vi "ExtPRFCount.vi"(0 "Therapy Delay (ms)":dbl=1.0 min=2.5e-08 format="%.3f", 1 "Start Counter?":bool=TRUE, 9 "Divide prf by":i32=2, 11 "pulse width (s or cycles)":dbl=0.0001 min=2.5e-08 format="%.2e") -> (6 "Therapy Delay (ms) out":dbl format="%.2f", 15 "Divide prf out":i32=1)   [LabVIEW 2022 SP3]
uses:
  Motion Controllers/-MotionRoutines/MotionGlobals.vi
  <vilib>/DAQmx/create/channels.llb/DAQmx Create Channel (CO-Pulse Generation-Ticks).vi
  <vilib>/DAQmx/configure/timing.llb/DAQmx Timing (Implicit).vi
  Pulsers/PulserGlobals.vi
panel:
  out "pulse width (s or cycles) out":dbl format="%.2e"
  # "Indicates if counter 0 is is giving a 1-1 output pulse\n for each motor inpute or if it is generating a continous prf."
  # "Determines whether counter 1 is used to fire \ntherapy at some divided multiple of counter 0."
  # "Divide by two will stop unexpectadly because of the circuitry. Therefore can divide by\n1, then the next option is three"
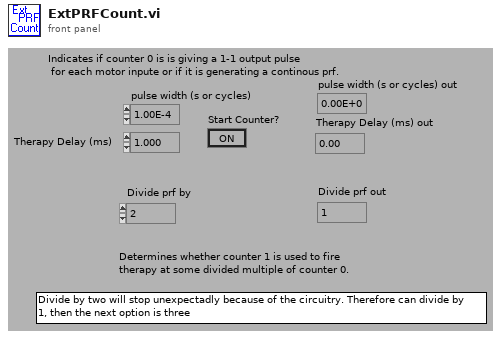
[diagram p1: front panel]
types:
  T1 = cluster{"Therapy frequency (MHz)":dbl, "Therapy amplitude (mV)":dbl, "time therapy on (s)":dbl, "Therapy Delay (ms) ":dbl, "Time (s)":dbl}
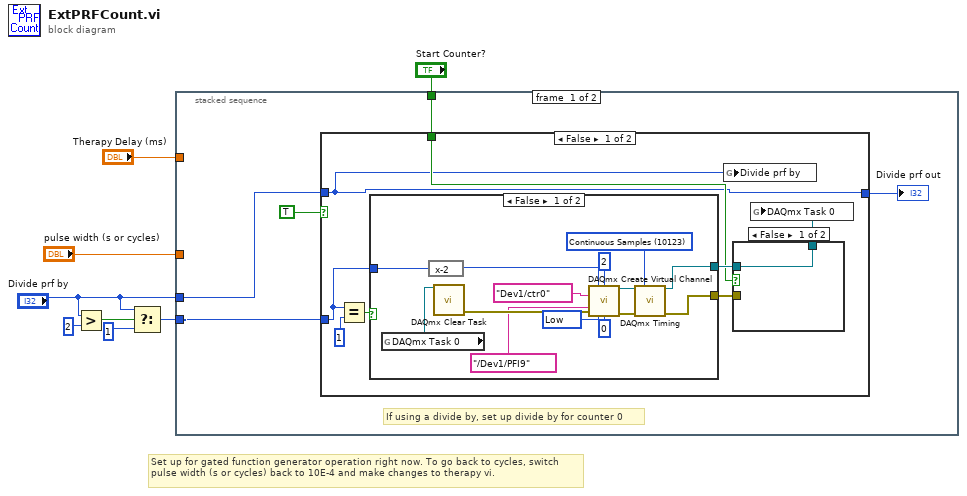
[diagram p0: block diagram]
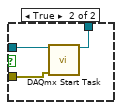
[diagram p2: hidden frame]
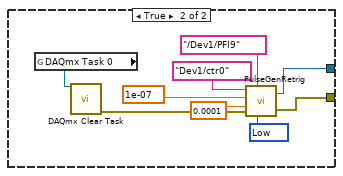
[diagram p3: hidden frame]
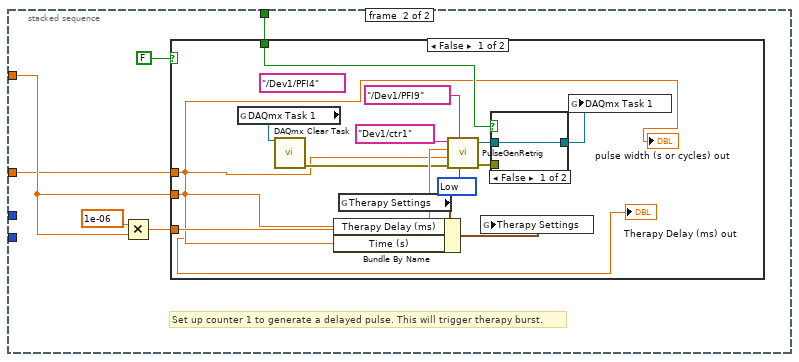
[diagram p5: hidden frame]
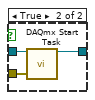
[diagram p6: hidden frame]
diagram:
  # "Set up for gated function generator operation right now. To go back to cycles, switch pulse width (s or cycles) back to 10E-4 and make changes to therapy vi."
  n1 = Greater?(x="Divide prf by", y=2) -> (0:w5:bool)
  n2 = Select(t="Divide prf by", s=w5, f=1) -> (s? t:f=w4:i32)
  n3 = stacked-sequence {
    tunnel: "Therapy Delay (ms)" -> [_ w54]
    tunnel: w4 -> [w12 _]
    tunnel: "Divide prf by" -> [w11 _]
    tunnel: "pulse width (s or cycles)" -> [_ w52]
    tunnel: "Start Counter?" -> [w9 w51]
    frame #0 {
      # "If using a divide by, set up divide by for counter 0"
      n4 = case shown="False" TRUE {
        tunnel: [w14 w49] -> w13
        tunnel: w11 -> [w14 _]
        tunnel: w12 -> [w19 w49]
        tunnel: w9 -> [w15 _]
        frame False {
          n5 = Equal?(x=w19, y=1) -> (x = y?=w20:bool)
          n6 = case shown="False" w20 {
            tunnel: w19 -> [w27 _]
            tunnel: [w39 w48] -> w18
            tunnel: [w38 w47] -> w17
            frame False {
              w29 = 10123 items=["Finite Samples"=10178, "Continuous Samples"=10123, "Hardware Timed Single Point"=12522] ("sample mode")
              w32 = 10214 items=["High"=10192, "Low"=10214] ("idle state")
              n7 = global read "MotionGlobals.vi" "DAQmx Task 0"() -> (w36:refnum<k21>)
              n8 = expression code="x-2"(w27) -> (w26:i32)
              n9 = call <vilib>:"DAQmx Clear Task.vi"("task in"=w36) -> ("error out"=w37:errorcluster)  [unwired: 1 in, 13 out]
              n10 = call-poly <vilib>:"DAQmx Create Virtual Channel.vi"("high ticks"=w26, "low ticks"=2, "counter"=tag "Dev1/ctr0", "source of ticks"=tag "/Dev1/PFI9", "error in"=w37, "idle state"=w32, "initial delay"=0) -> ("task out"=w31:refnum<k21>, "error out"=w30:errorcluster)  [unwired: 2 in, 5 out]
              n11 = call-poly <vilib>:"DAQmx Timing.vi"("task/channels in"=w31, "sample mode"=w29, "error in"=w30) -> ("task out"=w39:refnum<k21>, "error out"=w38:errorcluster)  [unwired: 1 in, 10 out]
            }
            frame True {
              w44 = 10214 items=["High"=10192, "Low"=10214] ("idle state")
              n12 = global read "MotionGlobals.vi" "DAQmx Task 0"() -> (w45:refnum<k21>)
              n13 = call <vilib>:"DAQmx Clear Task.vi"("task in"=w45) -> ("error out"=w46:errorcluster)  [unwired: 1 in, 13 out]
              n14 = call "PulseGenRetrig.vi"("idle state"=w44, "source"=tag "/Dev1/PFI9", "error in"=w46, "high time"=0.0001 ("pulse width (s or cycles)"), "pulse delay (s or cycles)"=1e-07, "counter"=tag "Dev1/ctr0") -> ("error out"=w47:errorcluster, "task out"=w48:refnum<k21>)
            }
          }
          n15 = global write "PulserGlobals.vi" "Divide prf by"(w14) -> ()
          n16 = case shown="False" w15 {
            tunnel: w18 -> [w22 w25]
            tunnel: w17 -> [_ w24]
            tunnel: [w22 w23] -> w16
            frame False {
            }
            frame True {
              n17 = call <vilib>:"DAQmx Start Task.vi"("task/channels in"=w25, "error in"=w24) -> ("task out"=w23:refnum<k21>)  [unwired: 13 out]
            }
          }
          n18 = global write "MotionGlobals.vi" "DAQmx Task 0"(w16) -> ()
        }
        frame True {
        }
      }
      "Divide prf out" <- w13
    }
    frame #1 {
      # "Set up counter 1 to generate a delayed pulse. This will trigger therapy burst."
      n19 = Multiply(x=1e-06 ("y"), y=w54) -> (x*y=w53:dbl)
      n20 = case shown="False" FALSE {
        tunnel: w53 -> [w69 _]
        tunnel: w54 -> [w56 _]
        tunnel: w52 -> [w57 _]
        tunnel: w51 -> [w68 _]
        frame False {
          (unwired) tag "/Dev1/PFI4" ("source")
          w63 = 10214 items=["High"=10192, "Low"=10214] ("idle state")
          n21 = global read "MotionGlobals.vi" "DAQmx Task 1"() -> (w66:refnum<k21>)
          n22 = call <vilib>:"DAQmx Clear Task.vi"("task in"=w66) -> ("error out"=w67:errorcluster)  [unwired: 1 in, 13 out]
          n23 = global read "PulserGlobals.vi" "Therapy Settings"() -> (w58:T1)
          n24 = Bundle By Name(cluster=w58, "Therapy Delay (ms)"=w56, "Time (s)"=w57) -> (w59:T1)
          n25 = call "PulseGenRetrig.vi"("idle state"=w63, "source"=tag "/Dev1/PFI9", "error in"=w67, "high time"=w57, "pulse delay (s or cycles)"=w69, "counter"=tag "Dev1/ctr1") -> ("error out"=w61:errorcluster, "task out"=w62:refnum<k21>)
          n26 = global write "PulserGlobals.vi" "Therapy Settings"(w59) -> ()
          n27 = case shown="False" w68 {
            tunnel: w62 -> [w70 w73]
            tunnel: w61 -> [_ w72]
            tunnel: [w70 w71] -> w60
            frame False {
            }
            frame True {
              n28 = call <vilib>:"DAQmx Start Task.vi"("task/channels in"=w73, "error in"=w72) -> ("task out"=w71:refnum<k21>)  [unwired: 13 out]
            }
          }
          n29 = global write "MotionGlobals.vi" "DAQmx Task 1"(w60) -> ()
          "Therapy Delay (ms) out" <- w56
          "pulse width (s or cycles) out" <- w57
        }
        frame True {
        }
      }
    }
  }
